vi "String - Get Dates.vi"(10 "End Date":timestamp format="%<%d/%m/%Y>T", 11 "Start Date":timestamp format="%<%d/%m/%Y>T") -> (2 "Total (Including Start Date)":i32, 3 "List of Dates YYYYmmDD":string[](array[string]))   [LabVIEW 2013]
panel:
  out "Days":dbl
  # "To"
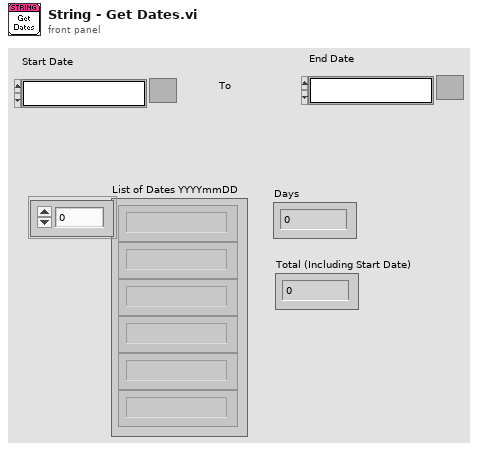
[diagram p1: front panel]
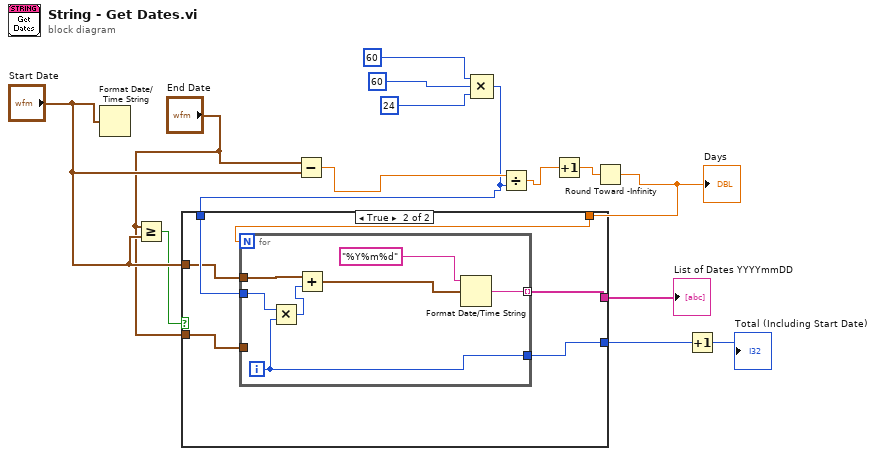
[diagram p0: block diagram]
diagram:
  n1 = Format Date/Time String(seconds (now)="Start Date") -> ()  [unwired: 2 in, 1 out]
  n2 = Greater Or Equal?(x="End Date", y="Start Date") -> (x >= y?=w8:bool)
  n3 = Subtract(x="End Date", y="Start Date") -> (x-y=w11:dbl)
  n4 = Compound Arithmetic op=MULTIPLY(60, 60 ("y"), 24 ("y")) -> (w10:i32)
  n5 = Divide(x=w11, y=w10) -> (x/y=w3:dbl)
  n6 = Increment(x=w3) -> (x+1=w1:dbl)
  n7 = Round Toward -Infinity(1:w1) -> (0:w2:dbl)
  "Days" <- w2
  n8 = case shown="True" w8 {
    tunnel: w10 -> [_ w20]
    tunnel: "Start Date" -> [_ w19]
    tunnel: "End Date" -> [_ w18]
    tunnel: [_ w17] -> w6
    tunnel: [_ w16] -> w5
    tunnel: w2 -> [_ w15]
    frame False {
    }
    frame True {
      n9 = for {
        N: w15 -> [_]
        tunnel: w19 -> [w27]
        tunnel: w20 -> [w22]
        tunnel: w18 -> [_]
        tunnel: [w24] -> w17 mode=indexing
        tunnel: [w23] -> w16
        i -> [w23]
        n10 = Multiply(x=w22, y=w23) -> (x*y=w21:i32)
        n11 = Add(x=w27, y=w21) -> (x+y=w26:timestamp)
        n12 = Format Date/Time String(time format string (%c)="%Y%m%d", seconds (now)=w26) -> (date/time string=w24:string)  [unwired: 1 in]
      }
    }
  }
  "List of Dates YYYYmmDD" <- w6
  n13 = Increment(x=w5) -> (x+1=→"Total (Including Start Date)":i32)
